vi "Ballard 429 - Clean-up.vi"(8 "Error (in)":errorcluster, 11 "Card Parameters (in)":T1) -> (0 "Error (out)":errorcluster)   [LabVIEW 2020, in "Ballard Arinc-429 Engine.lvlib"]
uses:
  Ballard Arinc-429 Engine.lvlib
  RT Controls/Card Parameters.ctl
  Shared/Controls and Global/Initialization Method.ctl
  <instrlib>/BTICardLib/BTICardLV.lvlib
  <instrlib>/BTI429Lib/BTI429LV.lvlib
  Shared/Ballard Arinc-429 Shared.lvlib
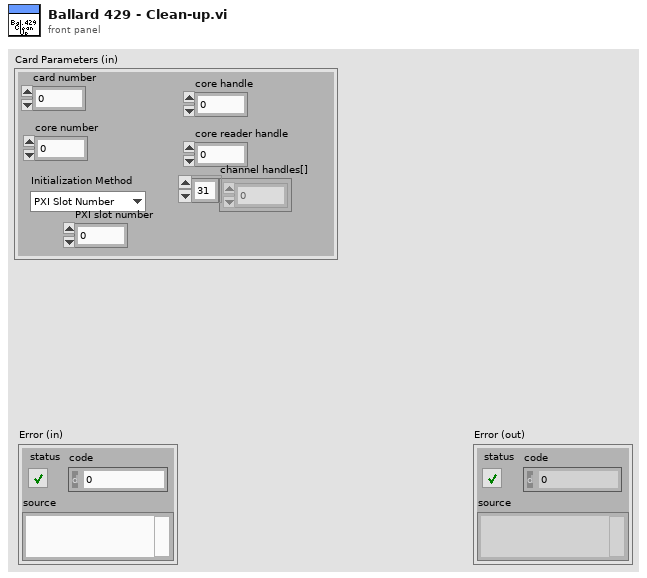
[diagram p1: front panel]
types:
  T1 = typedef "Ballard Arinc-429 Engine.lvlib/Card Parameters.ctl" = cluster{"card number":i32, "core number":i32, "core handle":u64, "core reader handle":u64, "channel handles[]":u64[], "Initialization Method":T2, "PXI slot number":i32}
  T2 = typedef "Ballard Arinc-429 Shared.lvlib/Initialization Method.ctl" = enum16{"PXI Slot Number", "Card Number"}
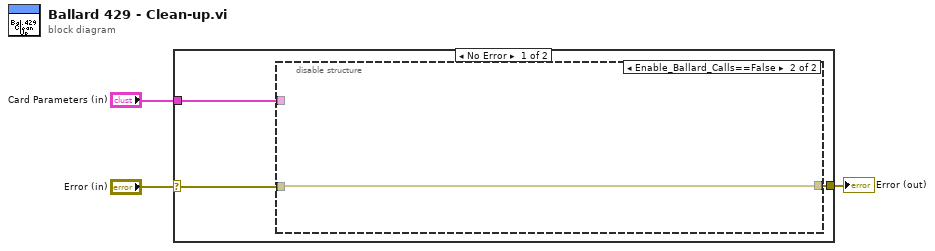
[diagram p0: block diagram]
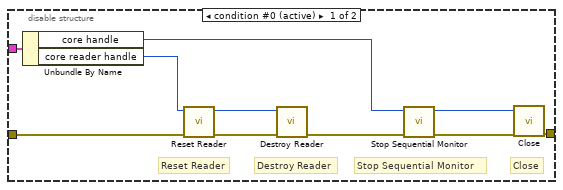
[diagram p2: hidden frame]
diagram:
  n1 = case shown="No Error" "Error (in)" {
    selector: "Error (in)" -> [w4 w18]
    tunnel: "Card Parameters (in)" -> [w6 _]
    tunnel: [w5 w18] -> w2
    frame No Error {
      n2 = disable-structure shown="Enable_Ballard_Calls==False" {
        disable-tunnel: w6 -> [w14 _]
        disable-tunnel: [w11 w17] -> w5
        disable-tunnel: w4 -> [w7 w17]
        frame condition #0 (active) {
          # "Destroy Reader"
          # "Close"
          # "Stop Sequential Monitor"
          # "Reset Reader"
          n3 = Unbundle By Name(w14) -> ("core handle"=w12:u64, "core reader handle"=w13:u64)
          n4 = call <instrlib>:"Reset Reader.vi"("error in (no error)"=w7, "reader handle in"=w13) -> ("error out"=w10:errorcluster, "reader handle out"=w8:u64)  [unwired: 8 in]
          n5 = call <instrlib>:"Destroy Reader.vi"("error in (no error)"=w10, "reader handle in"=w8) -> ("error out"=w9:errorcluster)  [unwired: 9 in]
          n6 = call <instrlib>:"Stop Sequential Monitor.vi"("error in (no error)"=w9, "core handle in"=w12) -> ("error out"=w15:errorcluster, "core handle out"=w16:u64)  [unwired: 8 in]
          n7 = call <instrlib>:"Close.vi"("error in (no error)"=w15, "core handle in"=w16) -> ("error out"=w11:errorcluster)  [unwired: 8 in, 1 out]
        }
        frame condition #1 {
        }
      }
    }
    frame Error {
    }
  }
  "Error (out)" <- w2
